vi "Terminal-SelfCheck-DAQCheck.vi"(9 "6220":T2, 10 "6133":T1, 11 "检验次数（5）":i32) -> (3 "结果":bool)   [LabVIEW 2014]
panel:
  out "轴向油缸力":sgl[](array[numeric])
  out "径向油缸力":sgl[](array[numeric])
  out "摩擦力2":sgl[](array[numeric])
  out "摩擦力1":sgl[](array[numeric])
  out "出油温度":sgl[](array[numeric])
  out "轴承外圈温度":sgl[](array[numeric])
  out "陪试轴承润滑单元出油温度2":sgl[](array[numeric])
  out "陪试轴承润滑单元出油温度1":sgl[](array[numeric])
  out "加速度2":sgl[](array[numeric])
  out "加速度1":sgl[](array[numeric])
  out "电涡流5":sgl[](array[numeric])
  out "电涡流4":sgl[](array[numeric])
  out "电涡流3":sgl[](array[numeric])
  out "电涡流2":sgl[](array[numeric])
  out "电涡流1":sgl[](array[numeric])
  out "声发射":sgl[](array[numeric])
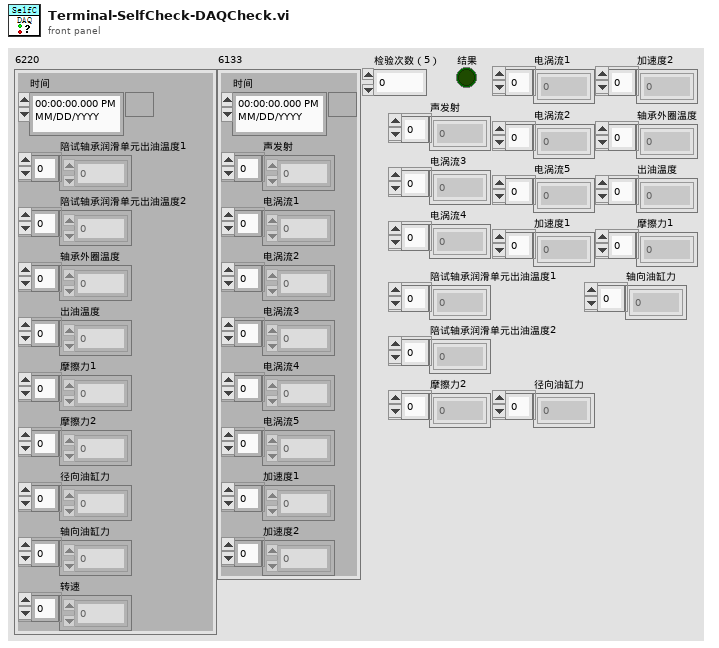
[diagram p1: front panel]
types:
  T1 = cluster{"时间":timestamp, "声发射":sgl[], "电涡流1":sgl[], "电涡流2":sgl[], "电涡流3":sgl[], "电涡流4":sgl[], "电涡流5":sgl[], "加速度1":sgl[], "加速度2":sgl[]}
  T2 = cluster{"时间":timestamp, "陪试轴承润滑单元出油温度1":sgl[], "陪试轴承润滑单元出油温度2":sgl[], "轴承外圈温度":sgl[], "出油温度":sgl[], "摩擦力1":sgl[], "摩擦力2":sgl[], "径向油缸力":sgl[], "轴向油缸力":sgl[], "转速":sgl[]}
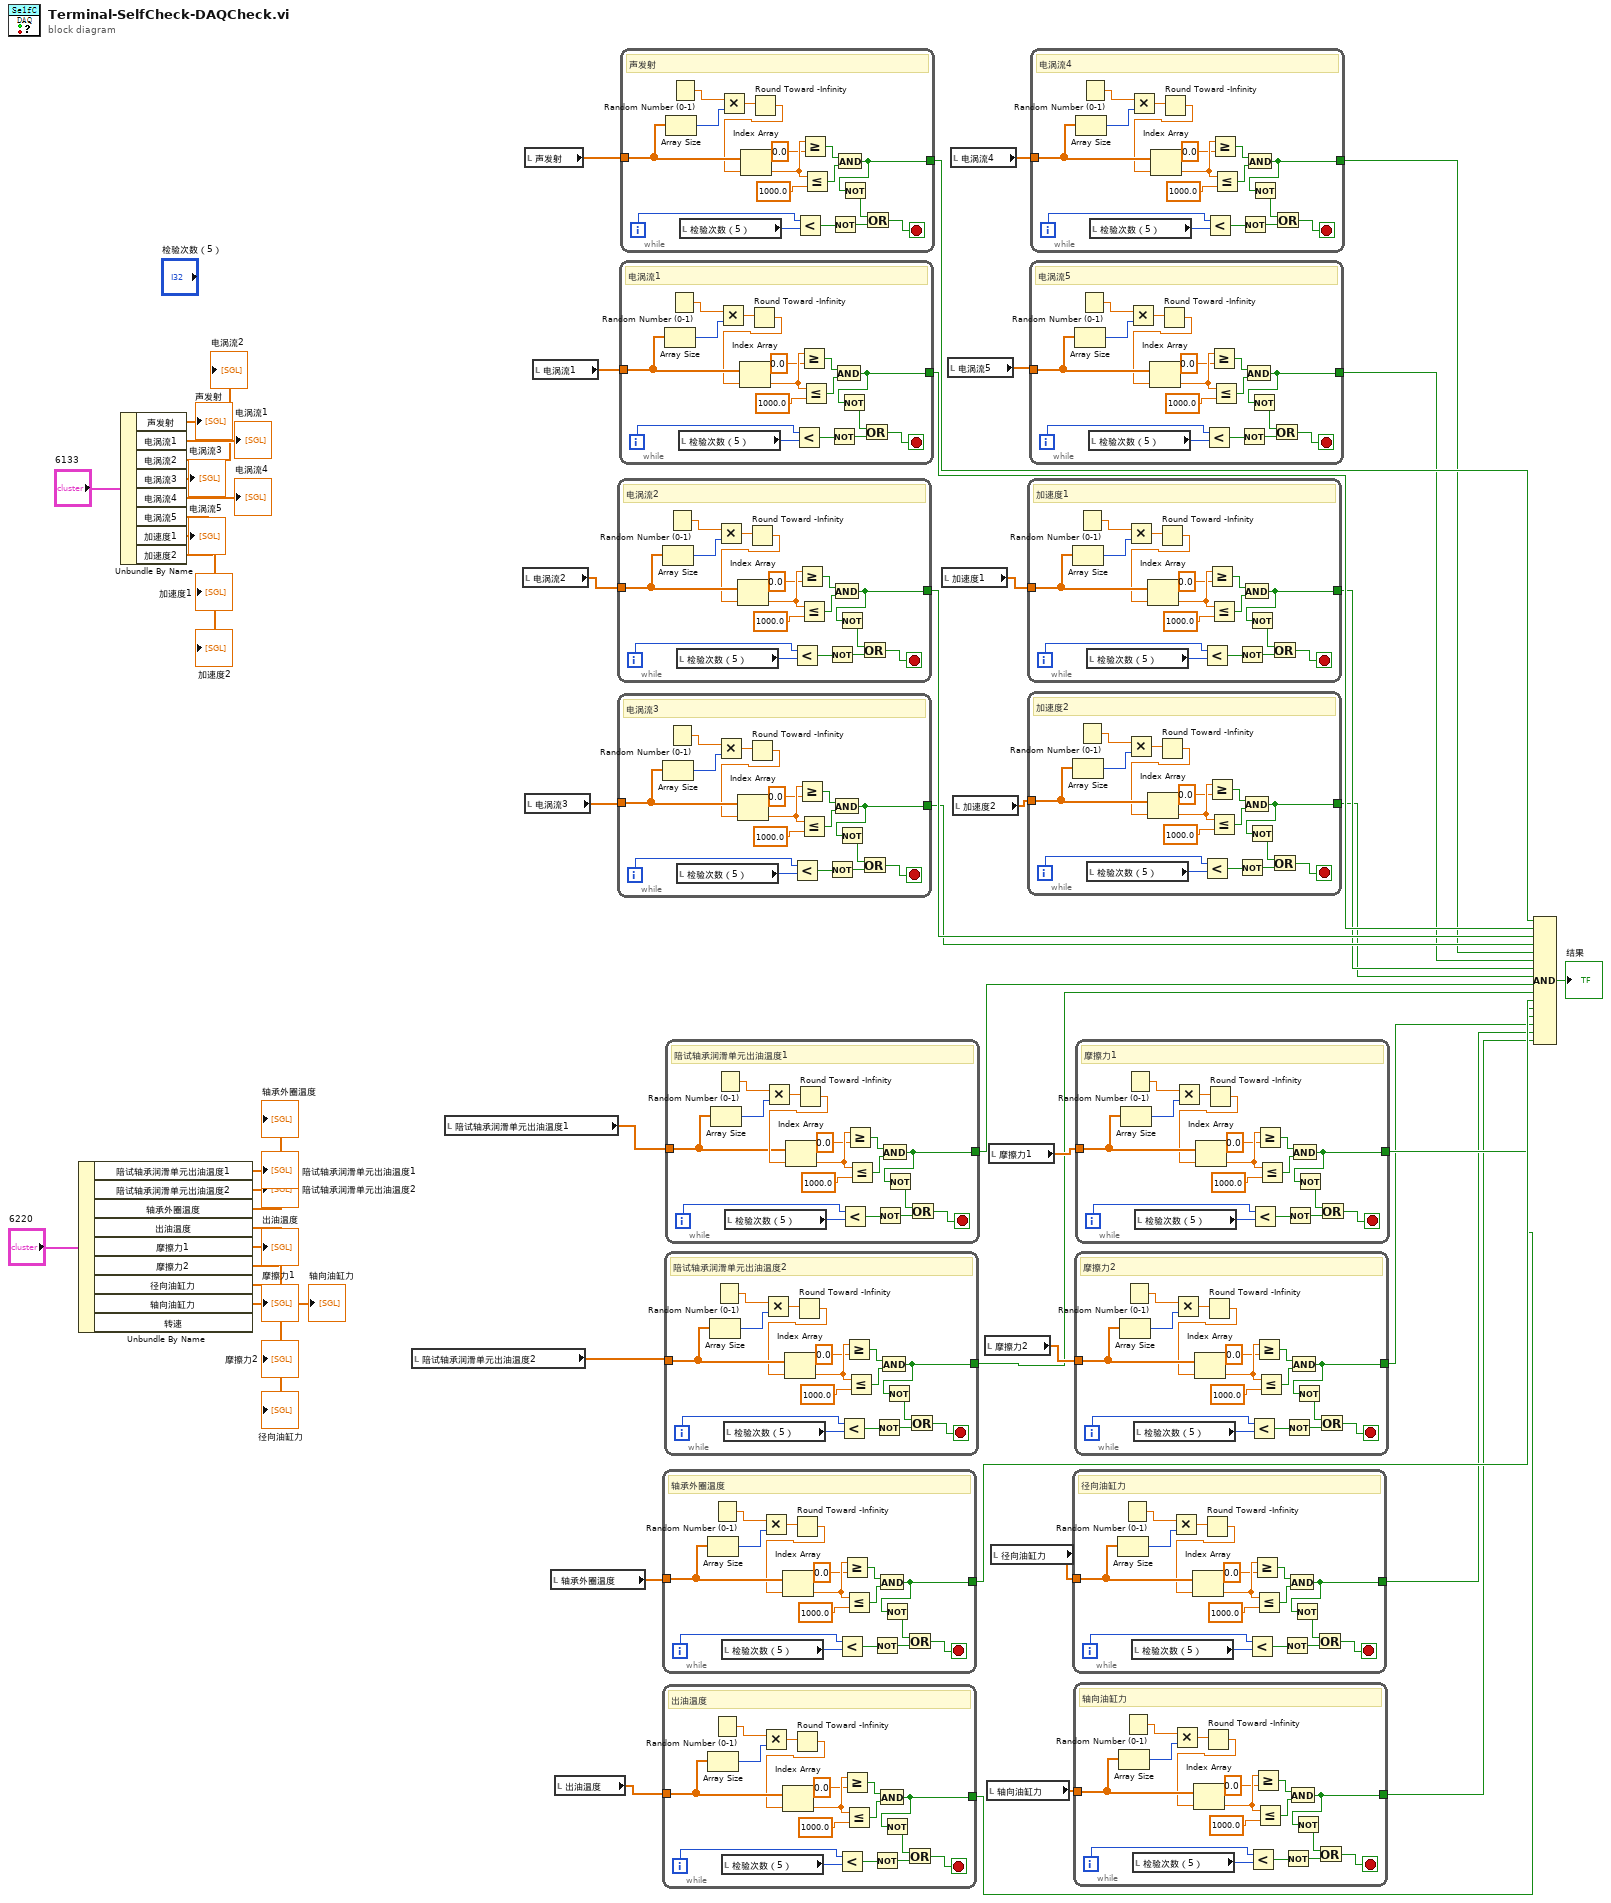
[diagram p0: block diagram]
diagram:
  n1 = Unbundle By Name("6220") -> ("陪试轴承润滑单元出油温度1"=→"陪试轴承润滑单元出油温度1":sgl[], "陪试轴承润滑单元出油温度2"=→"陪试轴承润滑单元出油温度2":sgl[], "轴承外圈温度"=→"轴承外圈温度":sgl[], "出油温度"=→"出油温度":sgl[], "摩擦力1"=→"摩擦力1":sgl[], "摩擦力2"=→"摩擦力2":sgl[], "径向油缸力"=→"径向油缸力":sgl[], "轴向油缸力"=→"轴向油缸力":sgl[])  [unwired: 1 out]
  n2 = Unbundle By Name("6133") -> ("声发射"=→"声发射":sgl[], "电涡流1"=→"电涡流1":sgl[], "电涡流2"=→"电涡流2":sgl[], "电涡流3"=→"电涡流3":sgl[], "电涡流4"=→"电涡流4":sgl[], "电涡流5"=→"电涡流5":sgl[], "加速度1"=→"加速度1":sgl[], "加速度2"=→"加速度2":sgl[])
  n3 = local read "陪试轴承润滑单元出油温度2"() -> (w24:sgl[])
  n4 = local read "陪试轴承润滑单元出油温度1"() -> (w25:sgl[])
  n5 = local read "电涡流2"() -> (w31:sgl[])
  n6 = local read "声发射"() -> (w41:sgl[])
  n7 = local read "电涡流3"() -> (w30:sgl[])
  n8 = local read "电涡流1"() -> (w40:sgl[])
  n9 = local read "轴承外圈温度"() -> (w23:sgl[])
  n10 = local read "出油温度"() -> (w22:sgl[])
  n11 = while {
    tunnel: w31 -> [w68]
    tunnel: [w52] -> w15
    i -> [w57]
    stop <- w54 stop-if-true
    # "电涡流2"
    n12 = Array Size(array=w68) -> (size(s)=w66:i32)
    n13 = Random Number (0-1)() -> (number: 0 to 1=w67:dbl)
    n14 = local read "检验次数（5）"() -> (w58:i32)
    n15 = Multiply(x=w67, y=w66) -> (x*y=w65:dbl)
    n16 = Round Toward -Infinity(1:w65) -> (0:w64:dbl)
    n17 = Index Array(array=w68, index=w64) -> (element=w63:sgl)
    n18 = Less?(x=w57, y=w58) -> (x < y?=w56:bool)
    n19 = Greater Or Equal?(x=w63, y=sgl 0.0) -> (x >= y?=w60:bool)
    n20 = Less Or Equal?(x=w63, y=sgl 1000.0) -> (x <= y?=w59:bool)
    n21 = Not(x=w56) -> (.not. x?=w55:bool)
    n22 = And(x=w60, y=w59) -> (x .and. y?=w52:bool)
    n23 = Not(x=w52) -> (.not. x?=w53:bool)
    n24 = Or(x=w53, y=w55) -> (x .or. y?=w54:bool)
  }
  n25 = while {
    tunnel: w30 -> [w85]
    tunnel: [w69] -> w14
    i -> [w74]
    stop <- w71 stop-if-true
    # "电涡流3"
    n26 = Array Size(array=w85) -> (size(s)=w83:i32)
    n27 = Random Number (0-1)() -> (number: 0 to 1=w84:dbl)
    n28 = local read "检验次数（5）"() -> (w75:i32)
    n29 = Multiply(x=w84, y=w83) -> (x*y=w82:dbl)
    n30 = Round Toward -Infinity(1:w82) -> (0:w81:dbl)
    n31 = Index Array(array=w85, index=w81) -> (element=w80:sgl)
    n32 = Less?(x=w74, y=w75) -> (x < y?=w73:bool)
    n33 = Greater Or Equal?(x=w80, y=sgl 0.0) -> (x >= y?=w77:bool)
    n34 = Less Or Equal?(x=w80, y=sgl 1000.0) -> (x <= y?=w76:bool)
    n35 = Not(x=w73) -> (.not. x?=w72:bool)
    n36 = And(x=w77, y=w76) -> (x .and. y?=w69:bool)
    n37 = Not(x=w69) -> (.not. x?=w70:bool)
    n38 = Or(x=w70, y=w72) -> (x .or. y?=w71:bool)
  }
  n39 = while {
    tunnel: w40 -> [w102]
    tunnel: [w86] -> w16
    i -> [w91]
    stop <- w88 stop-if-true
    # "电涡流1"
    n40 = Array Size(array=w102) -> (size(s)=w100:i32)
    n41 = Random Number (0-1)() -> (number: 0 to 1=w101:dbl)
    n42 = local read "检验次数（5）"() -> (w92:i32)
    n43 = Multiply(x=w101, y=w100) -> (x*y=w99:dbl)
    n44 = Round Toward -Infinity(1:w99) -> (0:w98:dbl)
    n45 = Index Array(array=w102, index=w98) -> (element=w97:sgl)
    n46 = Less?(x=w91, y=w92) -> (x < y?=w90:bool)
    n47 = Greater Or Equal?(x=w97, y=sgl 0.0) -> (x >= y?=w94:bool)
    n48 = Less Or Equal?(x=w97, y=sgl 1000.0) -> (x <= y?=w93:bool)
    n49 = Not(x=w90) -> (.not. x?=w89:bool)
    n50 = And(x=w94, y=w93) -> (x .and. y?=w86:bool)
    n51 = Not(x=w86) -> (.not. x?=w87:bool)
    n52 = Or(x=w87, y=w89) -> (x .or. y?=w88:bool)
  }
  n53 = while {
    tunnel: w41 -> [w119]
    tunnel: [w103] -> w17
    i -> [w108]
    stop <- w105 stop-if-true
    # "声发射"
    n54 = Array Size(array=w119) -> (size(s)=w117:i32)
    n55 = Random Number (0-1)() -> (number: 0 to 1=w118:dbl)
    n56 = local read "检验次数（5）"() -> (w109:i32)
    n57 = Multiply(x=w118, y=w117) -> (x*y=w116:dbl)
    n58 = Round Toward -Infinity(1:w116) -> (0:w115:dbl)
    n59 = Index Array(array=w119, index=w115) -> (element=w114:sgl)
    n60 = Less?(x=w108, y=w109) -> (x < y?=w107:bool)
    n61 = Greater Or Equal?(x=w114, y=sgl 0.0) -> (x >= y?=w111:bool)
    n62 = Less Or Equal?(x=w114, y=sgl 1000.0) -> (x <= y?=w110:bool)
    n63 = Not(x=w107) -> (.not. x?=w106:bool)
    n64 = And(x=w111, y=w110) -> (x .and. y?=w103:bool)
    n65 = Not(x=w103) -> (.not. x?=w104:bool)
    n66 = Or(x=w104, y=w106) -> (x .or. y?=w105:bool)
  }
  n67 = while {
    tunnel: w23 -> [w136]
    tunnel: [w120] -> w7
    i -> [w125]
    stop <- w122 stop-if-true
    # "轴承外圈温度"
    n68 = Array Size(array=w136) -> (size(s)=w134:i32)
    n69 = Random Number (0-1)() -> (number: 0 to 1=w135:dbl)
    n70 = local read "检验次数（5）"() -> (w126:i32)
    n71 = Multiply(x=w135, y=w134) -> (x*y=w133:dbl)
    n72 = Round Toward -Infinity(1:w133) -> (0:w132:dbl)
    n73 = Index Array(array=w136, index=w132) -> (element=w131:sgl)
    n74 = Less?(x=w125, y=w126) -> (x < y?=w124:bool)
    n75 = Greater Or Equal?(x=w131, y=sgl 0.0) -> (x >= y?=w128:bool)
    n76 = Less Or Equal?(x=w131, y=sgl 1000.0) -> (x <= y?=w127:bool)
    n77 = Not(x=w124) -> (.not. x?=w123:bool)
    n78 = And(x=w128, y=w127) -> (x .and. y?=w120:bool)
    n79 = Not(x=w120) -> (.not. x?=w121:bool)
    n80 = Or(x=w121, y=w123) -> (x .or. y?=w122:bool)
  }
  n81 = while {
    tunnel: w22 -> [w153]
    tunnel: [w137] -> w6
    i -> [w142]
    stop <- w139 stop-if-true
    # "出油温度"
    n82 = Array Size(array=w153) -> (size(s)=w151:i32)
    n83 = Random Number (0-1)() -> (number: 0 to 1=w152:dbl)
    n84 = local read "检验次数（5）"() -> (w143:i32)
    n85 = Multiply(x=w152, y=w151) -> (x*y=w150:dbl)
    n86 = Round Toward -Infinity(1:w150) -> (0:w149:dbl)
    n87 = Index Array(array=w153, index=w149) -> (element=w148:sgl)
    n88 = Less?(x=w142, y=w143) -> (x < y?=w141:bool)
    n89 = Greater Or Equal?(x=w148, y=sgl 0.0) -> (x >= y?=w145:bool)
    n90 = Less Or Equal?(x=w148, y=sgl 1000.0) -> (x <= y?=w144:bool)
    n91 = Not(x=w141) -> (.not. x?=w140:bool)
    n92 = And(x=w145, y=w144) -> (x .and. y?=w137:bool)
    n93 = Not(x=w137) -> (.not. x?=w138:bool)
    n94 = Or(x=w138, y=w140) -> (x .or. y?=w139:bool)
  }
  n95 = while {
    tunnel: w24 -> [w170]
    tunnel: [w154] -> w8
    i -> [w159]
    stop <- w156 stop-if-true
    # "陪试轴承润滑单元出油温度2"
    n96 = Array Size(array=w170) -> (size(s)=w168:i32)
    n97 = Random Number (0-1)() -> (number: 0 to 1=w169:dbl)
    n98 = local read "检验次数（5）"() -> (w160:i32)
    n99 = Multiply(x=w169, y=w168) -> (x*y=w167:dbl)
    n100 = Round Toward -Infinity(1:w167) -> (0:w166:dbl)
    n101 = Index Array(array=w170, index=w166) -> (element=w165:sgl)
    n102 = Less?(x=w159, y=w160) -> (x < y?=w158:bool)
    n103 = Greater Or Equal?(x=w165, y=sgl 0.0) -> (x >= y?=w162:bool)
    n104 = Less Or Equal?(x=w165, y=sgl 1000.0) -> (x <= y?=w161:bool)
    n105 = Not(x=w158) -> (.not. x?=w157:bool)
    n106 = And(x=w162, y=w161) -> (x .and. y?=w154:bool)
    n107 = Not(x=w154) -> (.not. x?=w155:bool)
    n108 = Or(x=w155, y=w157) -> (x .or. y?=w156:bool)
  }
  n109 = while {
    tunnel: w25 -> [w171]
    tunnel: [w172] -> w9
    i -> [w177]
    stop <- w174 stop-if-true
    # "陪试轴承润滑单元出油温度1"
    n110 = Array Size(array=w171) -> (size(s)=w186:i32)
    n111 = Random Number (0-1)() -> (number: 0 to 1=w187:dbl)
    n112 = local read "检验次数（5）"() -> (w178:i32)
    n113 = Multiply(x=w187, y=w186) -> (x*y=w185:dbl)
    n114 = Round Toward -Infinity(1:w185) -> (0:w184:dbl)
    n115 = Index Array(array=w171, index=w184) -> (element=w183:sgl)
    n116 = Less?(x=w177, y=w178) -> (x < y?=w176:bool)
    n117 = Greater Or Equal?(x=w183, y=sgl 0.0) -> (x >= y?=w180:bool)
    n118 = Less Or Equal?(x=w183, y=sgl 1000.0) -> (x <= y?=w179:bool)
    n119 = Not(x=w176) -> (.not. x?=w175:bool)
    n120 = And(x=w180, y=w179) -> (x .and. y?=w172:bool)
    n121 = Not(x=w172) -> (.not. x?=w173:bool)
    n122 = Or(x=w173, y=w175) -> (x .or. y?=w174:bool)
  }
  n123 = local read "加速度1"() -> (w27:sgl[])
  n124 = local read "电涡流5"() -> (w28:sgl[])
  n125 = local read "电涡流4"() -> (w29:sgl[])
  n126 = local read "加速度2"() -> (w26:sgl[])
  n127 = local read "摩擦力2"() -> (w20:sgl[])
  n128 = local read "轴向油缸力"() -> (w18:sgl[])
  n129 = local read "摩擦力1"() -> (w21:sgl[])
  n130 = local read "径向油缸力"() -> (w19:sgl[])
  n131 = while {
    tunnel: w27 -> [w204]
    tunnel: [w188] -> w11
    i -> [w193]
    stop <- w190 stop-if-true
    # "加速度1"
    n132 = Array Size(array=w204) -> (size(s)=w202:i32)
    n133 = Random Number (0-1)() -> (number: 0 to 1=w203:dbl)
    n134 = local read "检验次数（5）"() -> (w194:i32)
    n135 = Multiply(x=w203, y=w202) -> (x*y=w201:dbl)
    n136 = Round Toward -Infinity(1:w201) -> (0:w200:dbl)
    n137 = Index Array(array=w204, index=w200) -> (element=w199:sgl)
    n138 = Less?(x=w193, y=w194) -> (x < y?=w192:bool)
    n139 = Greater Or Equal?(x=w199, y=sgl 0.0) -> (x >= y?=w196:bool)
    n140 = Less Or Equal?(x=w199, y=sgl 1000.0) -> (x <= y?=w195:bool)
    n141 = Not(x=w192) -> (.not. x?=w191:bool)
    n142 = And(x=w196, y=w195) -> (x .and. y?=w188:bool)
    n143 = Not(x=w188) -> (.not. x?=w189:bool)
    n144 = Or(x=w189, y=w191) -> (x .or. y?=w190:bool)
  }
  n145 = while {
    tunnel: w26 -> [w221]
    tunnel: [w205] -> w10
    i -> [w210]
    stop <- w207 stop-if-true
    # "加速度2"
    n146 = Array Size(array=w221) -> (size(s)=w219:i32)
    n147 = Random Number (0-1)() -> (number: 0 to 1=w220:dbl)
    n148 = local read "检验次数（5）"() -> (w211:i32)
    n149 = Multiply(x=w220, y=w219) -> (x*y=w218:dbl)
    n150 = Round Toward -Infinity(1:w218) -> (0:w217:dbl)
    n151 = Index Array(array=w221, index=w217) -> (element=w216:sgl)
    n152 = Less?(x=w210, y=w211) -> (x < y?=w209:bool)
    n153 = Greater Or Equal?(x=w216, y=sgl 0.0) -> (x >= y?=w213:bool)
    n154 = Less Or Equal?(x=w216, y=sgl 1000.0) -> (x <= y?=w212:bool)
    n155 = Not(x=w209) -> (.not. x?=w208:bool)
    n156 = And(x=w213, y=w212) -> (x .and. y?=w205:bool)
    n157 = Not(x=w205) -> (.not. x?=w206:bool)
    n158 = Or(x=w206, y=w208) -> (x .or. y?=w207:bool)
  }
  n159 = while {
    tunnel: w28 -> [w238]
    tunnel: [w222] -> w12
    i -> [w227]
    stop <- w224 stop-if-true
    # "电涡流5"
    n160 = Array Size(array=w238) -> (size(s)=w236:i32)
    n161 = Random Number (0-1)() -> (number: 0 to 1=w237:dbl)
    n162 = local read "检验次数（5）"() -> (w228:i32)
    n163 = Multiply(x=w237, y=w236) -> (x*y=w235:dbl)
    n164 = Round Toward -Infinity(1:w235) -> (0:w234:dbl)
    n165 = Index Array(array=w238, index=w234) -> (element=w233:sgl)
    n166 = Less?(x=w227, y=w228) -> (x < y?=w226:bool)
    n167 = Greater Or Equal?(x=w233, y=sgl 0.0) -> (x >= y?=w230:bool)
    n168 = Less Or Equal?(x=w233, y=sgl 1000.0) -> (x <= y?=w229:bool)
    n169 = Not(x=w226) -> (.not. x?=w225:bool)
    n170 = And(x=w230, y=w229) -> (x .and. y?=w222:bool)
    n171 = Not(x=w222) -> (.not. x?=w223:bool)
    n172 = Or(x=w223, y=w225) -> (x .or. y?=w224:bool)
  }
  n173 = while {
    tunnel: w29 -> [w255]
    tunnel: [w239] -> w13
    i -> [w244]
    stop <- w241 stop-if-true
    # "电涡流4"
    n174 = Array Size(array=w255) -> (size(s)=w253:i32)
    n175 = Random Number (0-1)() -> (number: 0 to 1=w254:dbl)
    n176 = local read "检验次数（5）"() -> (w245:i32)
    n177 = Multiply(x=w254, y=w253) -> (x*y=w252:dbl)
    n178 = Round Toward -Infinity(1:w252) -> (0:w251:dbl)
    n179 = Index Array(array=w255, index=w251) -> (element=w250:sgl)
    n180 = Less?(x=w244, y=w245) -> (x < y?=w243:bool)
    n181 = Greater Or Equal?(x=w250, y=sgl 0.0) -> (x >= y?=w247:bool)
    n182 = Less Or Equal?(x=w250, y=sgl 1000.0) -> (x <= y?=w246:bool)
    n183 = Not(x=w243) -> (.not. x?=w242:bool)
    n184 = And(x=w247, y=w246) -> (x .and. y?=w239:bool)
    n185 = Not(x=w239) -> (.not. x?=w240:bool)
    n186 = Or(x=w240, y=w242) -> (x .or. y?=w241:bool)
  }
  n187 = while {
    tunnel: w19 -> [w272]
    tunnel: [w256] -> w3
    i -> [w261]
    stop <- w258 stop-if-true
    # "径向油缸力"
    n188 = Array Size(array=w272) -> (size(s)=w270:i32)
    n189 = Random Number (0-1)() -> (number: 0 to 1=w271:dbl)
    n190 = local read "检验次数（5）"() -> (w262:i32)
    n191 = Multiply(x=w271, y=w270) -> (x*y=w269:dbl)
    n192 = Round Toward -Infinity(1:w269) -> (0:w268:dbl)
    n193 = Index Array(array=w272, index=w268) -> (element=w267:sgl)
    n194 = Less?(x=w261, y=w262) -> (x < y?=w260:bool)
    n195 = Greater Or Equal?(x=w267, y=sgl 0.0) -> (x >= y?=w264:bool)
    n196 = Less Or Equal?(x=w267, y=sgl 1000.0) -> (x <= y?=w263:bool)
    n197 = Not(x=w260) -> (.not. x?=w259:bool)
    n198 = And(x=w264, y=w263) -> (x .and. y?=w256:bool)
    n199 = Not(x=w256) -> (.not. x?=w257:bool)
    n200 = Or(x=w257, y=w259) -> (x .or. y?=w258:bool)
  }
  n201 = while {
    tunnel: w18 -> [w289]
    tunnel: [w273] -> w2
    i -> [w278]
    stop <- w275 stop-if-true
    # "轴向油缸力"
    n202 = Array Size(array=w289) -> (size(s)=w287:i32)
    n203 = Random Number (0-1)() -> (number: 0 to 1=w288:dbl)
    n204 = local read "检验次数（5）"() -> (w279:i32)
    n205 = Multiply(x=w288, y=w287) -> (x*y=w286:dbl)
    n206 = Round Toward -Infinity(1:w286) -> (0:w285:dbl)
    n207 = Index Array(array=w289, index=w285) -> (element=w284:sgl)
    n208 = Less?(x=w278, y=w279) -> (x < y?=w277:bool)
    n209 = Greater Or Equal?(x=w284, y=sgl 0.0) -> (x >= y?=w281:bool)
    n210 = Less Or Equal?(x=w284, y=sgl 1000.0) -> (x <= y?=w280:bool)
    n211 = Not(x=w277) -> (.not. x?=w276:bool)
    n212 = And(x=w281, y=w280) -> (x .and. y?=w273:bool)
    n213 = Not(x=w273) -> (.not. x?=w274:bool)
    n214 = Or(x=w274, y=w276) -> (x .or. y?=w275:bool)
  }
  n215 = while {
    tunnel: w20 -> [w306]
    tunnel: [w290] -> w4
    i -> [w295]
    stop <- w292 stop-if-true
    # "摩擦力2"
    n216 = Array Size(array=w306) -> (size(s)=w304:i32)
    n217 = Random Number (0-1)() -> (number: 0 to 1=w305:dbl)
    n218 = local read "检验次数（5）"() -> (w296:i32)
    n219 = Multiply(x=w305, y=w304) -> (x*y=w303:dbl)
    n220 = Round Toward -Infinity(1:w303) -> (0:w302:dbl)
    n221 = Index Array(array=w306, index=w302) -> (element=w301:sgl)
    n222 = Less?(x=w295, y=w296) -> (x < y?=w294:bool)
    n223 = Greater Or Equal?(x=w301, y=sgl 0.0) -> (x >= y?=w298:bool)
    n224 = Less Or Equal?(x=w301, y=sgl 1000.0) -> (x <= y?=w297:bool)
    n225 = Not(x=w294) -> (.not. x?=w293:bool)
    n226 = And(x=w298, y=w297) -> (x .and. y?=w290:bool)
    n227 = Not(x=w290) -> (.not. x?=w291:bool)
    n228 = Or(x=w291, y=w293) -> (x .or. y?=w292:bool)
  }
  n229 = while {
    tunnel: w21 -> [w323]
    tunnel: [w307] -> w5
    i -> [w312]
    stop <- w309 stop-if-true
    # "摩擦力1"
    n230 = Array Size(array=w323) -> (size(s)=w321:i32)
    n231 = Random Number (0-1)() -> (number: 0 to 1=w322:dbl)
    n232 = local read "检验次数（5）"() -> (w313:i32)
    n233 = Multiply(x=w322, y=w321) -> (x*y=w320:dbl)
    n234 = Round Toward -Infinity(1:w320) -> (0:w319:dbl)
    n235 = Index Array(array=w323, index=w319) -> (element=w318:sgl)
    n236 = Less?(x=w312, y=w313) -> (x < y?=w311:bool)
    n237 = Greater Or Equal?(x=w318, y=sgl 0.0) -> (x >= y?=w315:bool)
    n238 = Less Or Equal?(x=w318, y=sgl 1000.0) -> (x <= y?=w314:bool)
    n239 = Not(x=w311) -> (.not. x?=w310:bool)
    n240 = And(x=w315, y=w314) -> (x .and. y?=w307:bool)
    n241 = Not(x=w307) -> (.not. x?=w308:bool)
    n242 = Or(x=w308, y=w310) -> (x .or. y?=w309:bool)
  }
  n243 = Compound Arithmetic op=AND(w17, w16, w15, w14, w13, w12, w11, w10, w9, w8, w7, w6, w5, w4, w3, w2) -> (→"结果":bool)
